vi "GetErrorMsgyes.vi"(4 "error in (no error)":errorcluster, 5 "Device Address In":i32, 6 "DeviceKey In":string, 7 "CmdLib In":refnum<k24>) -> (0 "error out":errorcluster, 1 "Device Address Out":i32, 2 "DeviceKey Out":string, 3 "CmdLib Out":refnum<k24>)   [LabVIEW 2021]
uses:
  C:/Program Files/New Focus/New Focus Picomotor Application/Samples/LabVIEW/Model 8742/LabVIEW 2009/CmdLib.dll
  Program Files/New Focus/New Focus Picomotor Application/Samples/LabVIEW/Model 8742/LabVIEW 2009/CmdLib.dll
panel:
  in  "message":string
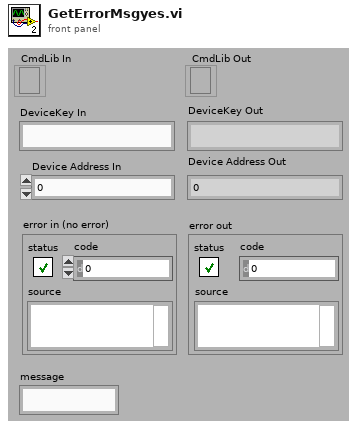
[diagram p1: front panel]
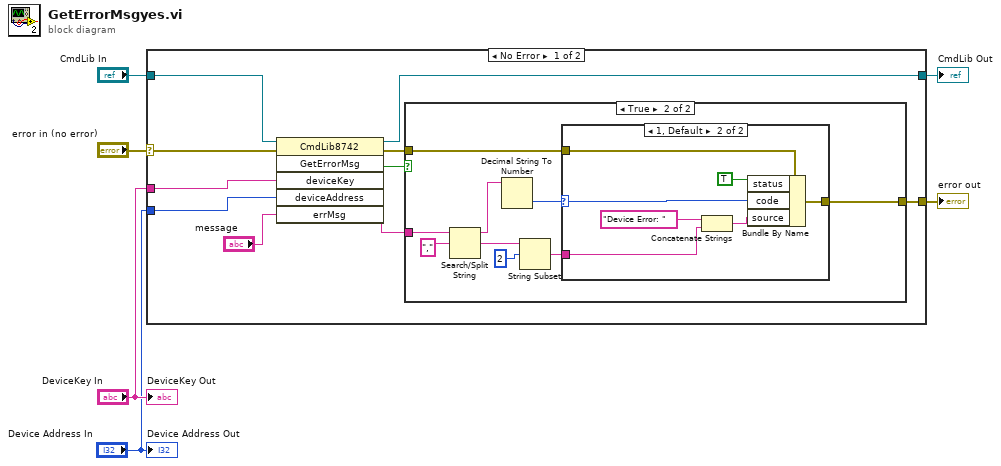
[diagram p0: block diagram]
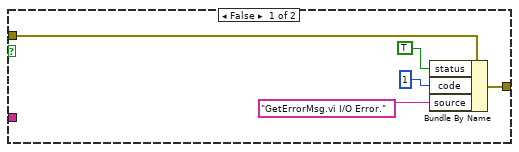
[diagram p2: hidden frame]
diagram:
  n1 = case shown="No Error" "error in (no error)" {
    selector: "error in (no error)" -> [w13 w39]
    tunnel: "CmdLib In" -> [w16 w40]
    tunnel: [w15 w40] -> w5
    tunnel: "DeviceKey In" -> [w14 _]
    tunnel: [w10 w39] -> w2
    tunnel: "Device Address In" -> [w8 _]
    frame No Error {
      n2 = invoke class="CmdLib8742" method="GetErrorMsg"(reference=w16, error in=w13, "deviceKey"=w14, "deviceAddress"=w8, "errMsg"="message") -> (reference out=w15:refnum<k24>, error out=w11:errorcluster, "GetErrorMsg"=w12:bool, "errMsg"=w7:string)  [unwired: 1 in, 2 out]
      n3 = case shown="True" w12 {
        tunnel: w11 -> [w21 w24]
        tunnel: [w20 w22] -> w10
        tunnel: w7 -> [_ w30]
        frame False {
          n4 = Bundle By Name(cluster=w21, "status"=TRUE, "code"=1, "source"="GetErrorMsg.vi I/O Error.") -> (w20:errorcluster)
        }
        frame True {
          n5 = Search/Split String(string=w30, search string/char (-)=",") -> (substring before match=w28:string, match + rest of string=w27:string)  [unwired: 1 in, 1 out]
          n6 = Decimal String To Number(string=w28) -> (number=w25:i32)  [unwired: 2 in, 1 out]
          n7 = String Subset(string=w27, offset (0)=2) -> (substring=w23:string)  [unwired: 1 in]
          n8 = case shown="1, Default" w25 {
            selector: w25 -> [_ w36]
            tunnel: w24 -> [w31 w37]
            tunnel: w23 -> [_ w34]
            tunnel: [w31 w35] -> w22
            frame 0 {
            }
            frame 1, Default {
              n9 = Concatenate Strings("Device Error: " ("string"), w34) -> (w33:string)
              n10 = Bundle By Name(cluster=w37, "status"=TRUE, "code"=w36, "source"=w33) -> (w35:errorcluster)
            }
          }
        }
      }
    }
    frame Error {
    }
  }
  "error out" <- w2
  "CmdLib Out" <- w5
  "DeviceKey Out" <- "DeviceKey In"
  "Device Address Out" <- "Device Address In"
